vi "RingsSub2.vi"(11 "Input depth":sgl[][](graph)=array540x960[518400 elements]) -> (1 "XY Graph 2":cluster{i32[], dbl[]}[](graph)=[{array[960 elements], array[960 elements]}, {[0, 1, 2, 3, 4, 5, 6, 7, 8, 9, 10, 11, 12, 13, 14, 15, 16, 17, 18, 19, 20, 21, 22, 23, 24, 25, 26, 27, 28, 29, 30, 31, 32, 33, 34, 35, 36, 37, 38, 39, 40, 41, 42, 43, 44, 45, 46, 47, 48, 49, 50, 51, 52, 53, 54, 55, 56, 57, 58, 59, 60, 61, 62, 63, 64, 65, 66, 67, 68, 69, 70, 71, 72, 73, 74, 75, 76, 77, 78, 79, 80, 81, 82, 83, 84, 85, 86, 87, 88, 89, 90, 91, 92, 93, 94, 95, 96, 97, 98, 99, 100, 101, 102, 103, 104, 105, 106, 107, 108, 109, 110, 111, 112, 113, 114, 115, 116, 117, 118, 119, 120, 121, 122, 123, 124, 125, 126, 127, 128, 129, 130, 131, 132, 133, 134, 135, 136, 137, 138, 139, 140, 141, 142, 143, 144, 145, 146, 147, 148, 149, 150, 151, 152, 153, 154, 155, 156, 157, 158, 159, 160, 161, 162, 163, 164, 165, 166, 167, 168, 169, 170, 171, 172, 173, 174, 175, 176, 177, 178, 179, 180, 181, 182, 183, 184, 185, 186, 187, 188, 189, 190, 191, 192, 193, 194, 195, 196, 197, 198, 199, 200, 201, 202, 203, 204, 205, 206, 207, 208, 209, 210, 211, 212, 213, 214, 215, 216, 217, 218, 219, 220, 221, 222, 223, 224, 225, 226, 227, 228, 229, 230, 231, 232, 233, 234, 235, 236, 237, 238, 239, 240, 241, 242, 243, 244, 245, 246, 247, 248, 249, 250, 251, 252, 253, 254, 255, 256, 257, 258, 259, 260, 261, 262, 263, 264, 265, 266, 267, 268, 269, 270, 271, 272, 273, 274, 275, 276, 277, 278, 279, 280, 281, 282, 283, 284, 285, 286, 287, 288, 289, 290, 291, 292, 293, 294, 295, 296, 297, 298, 299, 300, 301, 302, 303, 304, 305, 306, 307, 308, 309, 310, 311, 312, 313, 314, 315, 316, 317, 318, 319, 320, 321, 322, 323, 324, 325, 326, 327, 328, 329, 330, 331, 332, 333, 334, 335, 336, 337, 338, 339, 340, 341, 342, 343, 344, 345, 346, 347, 348, 349, 350, 351, 352, 353, 354, 355, 356, 357, 358, 359, 360, 361, 362, 363, 364, 365, 366, 367, 368, 369, 370, 371, 372, 373, 374, 375, 376, 377, 378, 379, 380, 381, 382, 383, 384, 385, 386, 387, 388, 389, 390, 391, 392, 393, 394, 395, 396, 397, 398, 399, 400, 401, 402, 403, 404, 405, 406, 407, 408, 409, 410, 411, 412, 413, 414, 415, 416, 417, 418, 419, 420, 421, 422, 423, 424, 425, 426, 427, 428, 429, 430, 431, 432, 433, 434, 435, 436, 437, 438, 439, 440, 441, 442, 443, 444, 445, 446, 447, 448, 449, 450, 451, 452, 453, 454, 455, 456, 457, 458, 459, 460, 461, 462, 463, 464, 465, 466, 467, 468, 469, 470, 471, 472, 473, 474, 475, 476, 477, 478, 479, 480, 481, 482, 483, 484, 485, 486, 487, 488, 489, 490, 491, 492, 493, 494, 495, 496, 497, 498, 499, 500, 501, 502, 503, 504, 505, 506, 507, 508, 509, 510, 511, 512, 513, 514, 515, 516, 517, 518, 519, 520, 521, 522, 523, 524, 525, 526, 527, 528, 529, 530, 531, 532, 533, 534, 535, 536, 537, 538, 539], array[540 elements]}], 2 "Peak-to-Peak, mm":sgl=16.549988, 3 "Tilt-Corrected depth":sgl[][](graph))   [LabVIEW 2017, in "libRealSense3.lvlib"]
uses:
  libRealSense3.lvlib
  <vilib>/Analysis/baseanly.llb/Mean (DBL).vi
  <vilib>/Analysis/NI_AALBase.lvlib
panel:
  out "index (row)":i32
  out "size(s) 2":i32=540
  out "x/y 2":sgl=960.0
  in  "Correct Y Tilt":bool=TRUE
  in  "Correct X tilt":bool=TRUE
  out "Numeric 2":sgl=913.3
  out "Numeric":sgl=909.3
  out "size(s)":i32[](array[numeric])=[540, 960]
  # "This Removes Tilt based on first and last values in X and Y. \n(It is strictly speaking NOT a plane fit)"
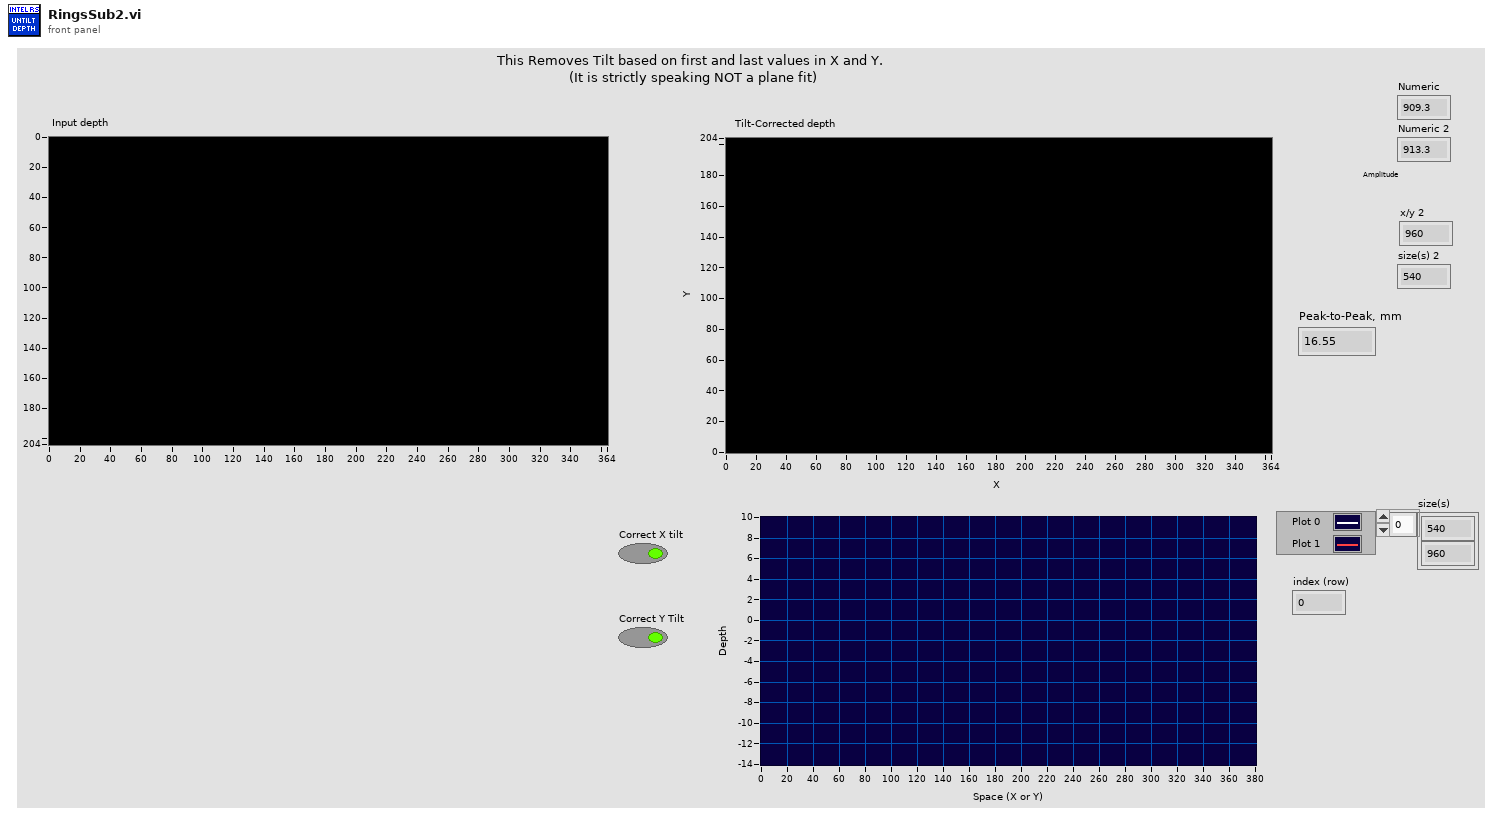
[diagram p1: front panel]
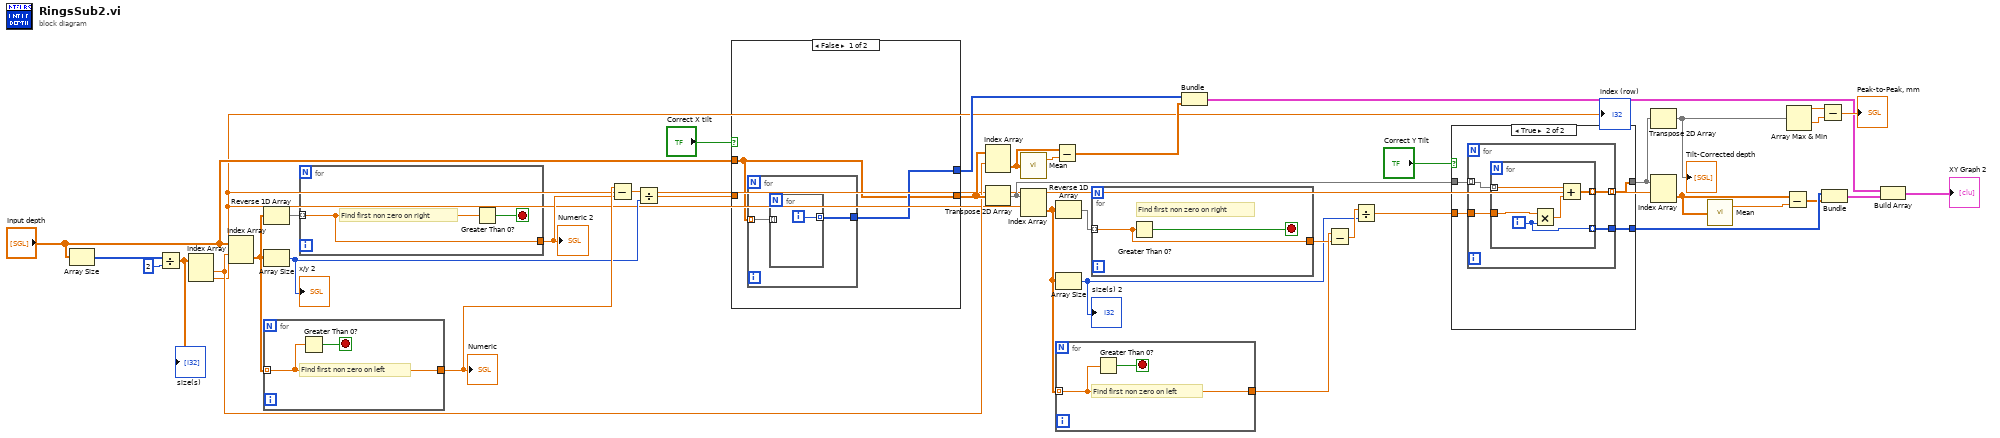
[diagram p0: block diagram]
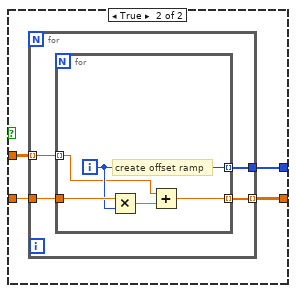
[diagram p3: hidden frame]
diagram:
  n1 = Array Size(array="Input depth") -> (size(s)=w11:i32[])
  n2 = Divide(x=w11, y=2) -> (x/y=w2:dbl[])
  "size(s)" <- w2
  n3 = Index Array(array=w2) -> (element #1=w8:dbl, element #2=w1:dbl)  [unwired: 2 in]
  "index (row)" <- w1
  n4 = Index Array(array="Input depth", index (row)=w8) -> (element=w12:sgl[])  [unwired: 1 in]
  n5 = Reverse 1D Array(array=w12) -> (reversed array=w32:sgl[])
  n6 = Array Size(array=w12) -> (size(s)=w5:i32)
  "x/y 2" <- w5
  n7 = for {
    tunnel: w12 -> [w42] mode=indexing
    tunnel: [w42] -> w33
    stop <- w41 stop-if-true
    # "Find first non zero on left"
    n8 = Greater Than 0?(x=w42) -> (x > 0?=w41:bool)
  }
  "Numeric" <- w33
  n9 = for {
    tunnel: w32 -> [w44] mode=indexing
    tunnel: [w44] -> w31
    stop <- w43 stop-if-true
    # "Find first non zero on right"
    n10 = Greater Than 0?(x=w44) -> (x > 0?=w43:bool)
  }
  "Numeric 2" <- w31
  n11 = Subtract(x=w33, y=w31) -> (x-y=w40:sgl)
  n12 = Divide(x=w40, y=w5) -> (x/y=w6:sgl)
  n13 = case shown="False" "Correct X tilt" {
    tunnel: w6 -> [_ w53]
    tunnel: [w45 w52] -> w26
    tunnel: [w46 w51] -> w24
    tunnel: "Input depth" -> [w45 w50]
    frame False {
      n14 = for {
        tunnel: [w48] -> w46
        tunnel: w45 -> [w47] mode=indexing
        n15 = for {
          tunnel: [w49] -> w48 mode=indexing
          tunnel: w47 -> [_] mode=indexing
          i -> [w49]
        }
      }
    }
    frame True {
      n16 = for {
        tunnel: w53 -> [w57]
        tunnel: w50 -> [w56] mode=indexing
        tunnel: [w55] -> w52 mode=indexing
        tunnel: [w54] -> w51
        n17 = for {
          tunnel: w56 -> [w59] mode=indexing
          tunnel: w57 -> [w62]
          tunnel: [w58] -> w55 mode=indexing
          tunnel: [w60] -> w54 mode=indexing
          i -> [w60]
          # "create offset ramp"
          n18 = Multiply(x=w62, y=w60) -> (x*y=w61:sgl)
          n19 = Add(x=w59, y=w61) -> (x+y=w58:sgl)
        }
      }
    }
  }
  n20 = Index Array(array=w26, index (row)=w8) -> (element=w15:sgl[])  [unwired: 1 in]
  n21 = Transpose 2D Array(2D array=w26) -> (transposed array=w34:sgl[][])
  n22 = call-poly <vilib>:"Mean.vi"("X"=w15) -> ("mean"=w16:dbl)  [unwired: 1 out]
  n23 = Index Array(array=w34, index (row)=w1) -> (element=w29:sgl[])  [unwired: 1 in]
  n24 = Subtract(x=w15, y=w16) -> (x-y=w14:dbl[])
  n25 = Reverse 1D Array(array=w29) -> (reversed array=w30:sgl[])
  n26 = Array Size(array=w29) -> (size(s)=w25:i32)
  "size(s) 2" <- w25
  n27 = for {
    tunnel: w29 -> [w64] mode=indexing
    tunnel: [w64] -> w28
    stop <- w63 stop-if-true
    # "Find first non zero on left"
    n28 = Greater Than 0?(x=w64) -> (x > 0?=w63:bool)
  }
  n29 = for {
    tunnel: w30 -> [w66] mode=indexing
    tunnel: [w66] -> w27
    stop <- w65 stop-if-true
    # "Find first non zero on right"
    n30 = Greater Than 0?(x=w66) -> (x > 0?=w65:bool)
  }
  n31 = Bundle(w24, w14) -> (w21:cluster{i32[], dbl[]})  [unwired: 1 in]
  n32 = Subtract(x=w28, y=w27) -> (x-y=w36:sgl)
  n33 = Divide(x=w36, y=w25) -> (x/y=w35:sgl)
  n34 = case shown="True" "Correct Y Tilt" {
    tunnel: w35 -> [_ w75]
    tunnel: w34 -> [w67 w74]
    tunnel: [w68 w73] -> w23
    tunnel: [w67 w72] -> w3
    frame False {
      n35 = for {
        tunnel: [w70] -> w68
        tunnel: w67 -> [w69] mode=indexing
        n36 = for {
          tunnel: [w71] -> w70 mode=indexing
          tunnel: w69 -> [_] mode=indexing
          i -> [w71]
        }
      }
    }
    frame True {
      n37 = for {
        tunnel: w75 -> [w79]
        tunnel: w74 -> [w78] mode=indexing
        tunnel: [w77] -> w72 mode=indexing
        tunnel: [w76] -> w73
        n38 = for {
          tunnel: w78 -> [w83] mode=indexing
          tunnel: w79 -> [w84]
          tunnel: [w81] -> w77 mode=indexing
          tunnel: [w80] -> w76 mode=indexing
          i -> [w80]
          n39 = Multiply(x=w84, y=w80) -> (x*y=w82:sgl)
          n40 = Add(x=w83, y=w82) -> (x+y=w81:sgl)
        }
      }
    }
  }
  n41 = Transpose 2D Array(2D array=w3) -> (transposed array=w4:sgl[][])
  "Tilt-Corrected depth" <- w4
  n42 = Index Array(array=w3, index (row)=w1) -> (element=w18:sgl[])  [unwired: 1 in]
  n43 = call-poly <vilib>:"Mean.vi"("X"=w18) -> ("mean"=w19:dbl)  [unwired: 1 out]
  n44 = Subtract(x=w18, y=w19) -> (x-y=w17:dbl[])
  n45 = Array Max & Min(array=w4) -> (max value=w39:sgl, min value=w38:sgl)  [unwired: 2 out]
  n46 = Subtract(x=w39, y=w38) -> (x-y=→"Peak-to-Peak, mm":sgl)
  n47 = Bundle(w23, w17) -> (w22:cluster{i32[], dbl[]})  [unwired: 1 in]
  n48 = Build Array(w21, w22) -> (→"XY Graph 2":cluster{i32[], dbl[]}[])
